vi "main_ctrl.vi"(8 "error in":errorcluster) -> (0 "error out":errorcluster caption="Error")   [LabVIEW 2013]
uses:
  <vilib>/Rock Robotics/WPI/DriverStation/WPI_DriverStationRobotMode2.ctl
  typedefs/fg_typedef.ctl
  typedefs/vision enable.ctl
  typedefs/vision data.ctl
  typedefs/subStates.ctl
  typedefs/singleUseSubstate.ctl
  <vilib>/Rock Robotics/WPI/Solenoid/WPI_SolenoidValue.ctl
  <vilib>/Rock Robotics/WPI/Compressor/WPI_CompressorGetSetRefNum.vi
  <vilib>/Rock Robotics/WPI/RobotDrive/WPI_RobotDriveGetSetRefNum.vi
  <vilib>/Rock Robotics/WPI/Solenoid/WPI_SolenoidSetEnum.vi
  <vilib>/Rock Robotics/WPI/RobotDrive/WPI_RobotDriveArcadeDrive_Standard(NoSaturation).vi
panel:
  out "Robot Mode":T1
  out "Vision SPI":u32
  out "Vision IPS":dbl
  out "Main IPS":dbl
  out "Main SPI":u32
  # "MAIN CONTROL"
  # "holds robot control code - dual parallel state machine"
  # "SPI: milliseconds per iteration\nIPS: iterations per second"
  # "need to incorporate cancel commands"
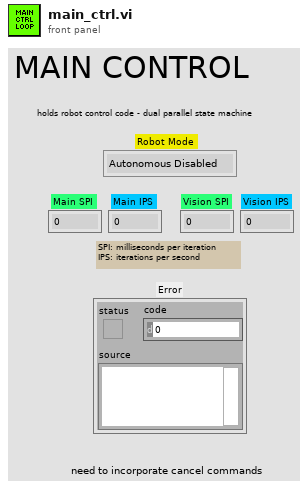
[diagram p1: front panel]
types:
  T1 = typedef "WPI_DriverStationRobotMode2.ctl" = enum16{"Autonomous Disabled", "Autonomous Enabled", "Teleop Disabled", "Teleop Enabled", "Timeout", "Finish", "Test Disabled", "Test Enabled"}
  T2 = typedef "vision data.ctl" = cluster{"x":dbl, "y":dbl, "area":dbl, "width":dbl, "height":dbl, "Hot Goal Present?":bool, "distance":dbl}
  T3 = typedef "vision enable.ctl" = enum16{"Enable", "Disable", "Stop"}
  T4 = typedef "fg_typedef.ctl" = enum16{"Get", "Set"}
  T5 = typedef "WPI_RobotDriveDevRef.ctl" = cluster{"DevStatus":errorcluster, "Motors[]":T6[], "Square Inputs":bool, "Max Output":dbl, "Isochronous":bool}
  T6 = typedef "WPI_MotorControlDeviceRef.ctl" = cluster{"DeviceStatus":errorcluster, "Type":enum16{"PWM", "CAN"}, "PWM":cluster{"Digital Module":T7, "PWM Channel":T8, "DeadBand":T9}, "CAN":cluster{"Device Number":u8, "Control Mode":T10, "Semaphore":T11, "Max Vout":dbl}, "Invert":bool, "TransformRef":T12, "InvTransformRef":T12}
  T7 = typedef "FPGA_TypedefDigitalModule.ctl" = enum16{"Digital Module 1", "Digital Module 2"}
  T8 = typedef "FPGA_DIOPWMChannel.ctl" = enum8{"PWM 1", "PWM 2", "PWM 3", "PWM 4", "PWM 5", "PWM 6", "PWM 7", "PWM 8", "PWM 9", "PWM 10", "Invalid"}
  T9 = typedef "WPI_PWMDeadband.ctl" = cluster{"Name":string, "maxPositivePwm":i32, "minPositivePwm":i32, "centerPwm":i32, "maxNegativePwm":i32, "minNegativePwm":i32, "angularRange":u16}
  T10 = typedef "WPI_CANJaguar_ControlMode.ctl" = enum8{"Percent VBus", "Current", "Speed", "Position", "Voltage"}
  T11 = typedef "Semaphore RefNum" = refnum<k1>
  T12 = typedef "WPI_PWMTransform_ConPane.ctl" = refnum<vi>
  T13 = typedef "WPI_SolenoidDevRef.ctl" = cluster{"DevStatus":errorcluster, "Solenoid Module":T14, "Forward Solenoid Channel":T15, "Reverse Solenoid Channel":T15}
  T14 = typedef "FPGA_TypedefSolenoidModule.ctl" = enum16{"Solenoid Module 1", "Solenoid Module 2"}
  T15 = typedef "WPI_SolenoidChannel.ctl" = enum8{"Solenoid 1", "Solenoid 2", "Solenoid 3", "Solenoid 4", "Solenoid 5", "Solenoid 6", "Solenoid 7", "Solenoid 8", "Invalid"}
  T16 = typedef "WPI_CompressorDevRef.ctl" = cluster{"DevStatus":errorcluster, "DigitalInputDevRef":T17, "RelayDevRef":T19}
  T17 = typedef "WPI_DigitalInputDevRef.ctl" = cluster{"DevStatus":errorcluster, "DIO Channel":T18, "Digital Module":T7}
  T18 = typedef "FPGA_DIOChannel.ctl" = enum8{"DIO 1", "DIO 2", "DIO 3", "DIO 4", "DIO 5", "DIO 6", "DIO 7", "DIO 8", "DIO 9", "DIO 10", "DIO 11", "DIO 12", "DIO 13", "DIO 14", "Invalid"}
  T19 = typedef "WPI_RelayDevRef.ctl" = cluster{"DevStatus":errorcluster, "Relay Channel":T20, "Digital Module":T7, "Relay Direction":T21}
  T20 = typedef "FPGA_DIORelayChannel.ctl" = enum8{"Relay 1", "Relay 2", "Relay 3", "Relay 4", "Relay 5", "Relay 6", "Relay 7", "Relay 8", "Invalid"}
  T21 = typedef "WPI_RelayDirection.ctl" = enum16{"Both directions", "Forward only", "Reverse only"}
  T22 = typedef "WPI_CameraDevRef.ctl" = cluster{"Camera Address":string, "CameraStatus":errorcluster, "Acquire Image Notifier":refnum<notifier>}
  T23 = typedef "IMAQ Image.ctl" = refnum<image>
  T24 = typedef "WPI_SolenoidValue.ctl" = enum16{"Off", "On", "Forward", "Reverse"}
  T25 = typedef "singleUseSubstate.ctl" = enum16{"null", "wait", "shift high", "shift low"}
  T26 = typedef "WPI_DriverStationDerivedRobotMode.ctl" = enum16{"Init", "Execute", "Stop"}
  T27 = typedef "subStates.ctl" = enum16{"null", "wait", "driver control", "auto", "manual override", "hold position", "rotate", "pickup", "pass", "load", "goto shoot", "shoot", "cancel", "end"}
  T28 = typedef "Loop 2 Datatype.ctl" = cluster{"State":T27, "Waiting Loop":i32, "State to Wait For":i32, "Loop ID":i32, "Exit Value":i32, "Joystick Y":dbl, "Tune Speed":dbl}
  T29 = typedef "Loop 1 Datatype.ctl" = cluster{"State":T27, "Waiting Loop":i32, "State to Wait For":i32, "Loop ID":i32, "Exit Value":i32}
  T30 = typedef "Loop 3 Datatype.ctl" = cluster{"State":T27, "Waiting Loop":i32, "State to Wait For":i32, "Loop ID":i32, "Exit Value":i32, "Joystick Y":dbl, "Joystick Z":dbl}
  T31 = typedef "Loop 0 Datatype.ctl" = cluster{"State":T27, "Waiting Loop":i32, "State to Wait For":i32, "Loop ID":i32, "Exit Value":i32, "X Axis":dbl, "Y Axis":dbl, "Z Axis":dbl}
  T32 = typedef "Loop 4 Datatype.ctl" = cluster{"State":T27, "Waiting Loop":i32, "State to Wait For":i32, "Loop ID":i32, "Exit Value":i32}
  T33 = cluster{"Vision mSPI":u32, "Main mSPI":u32, "Dash mSPI":u32}
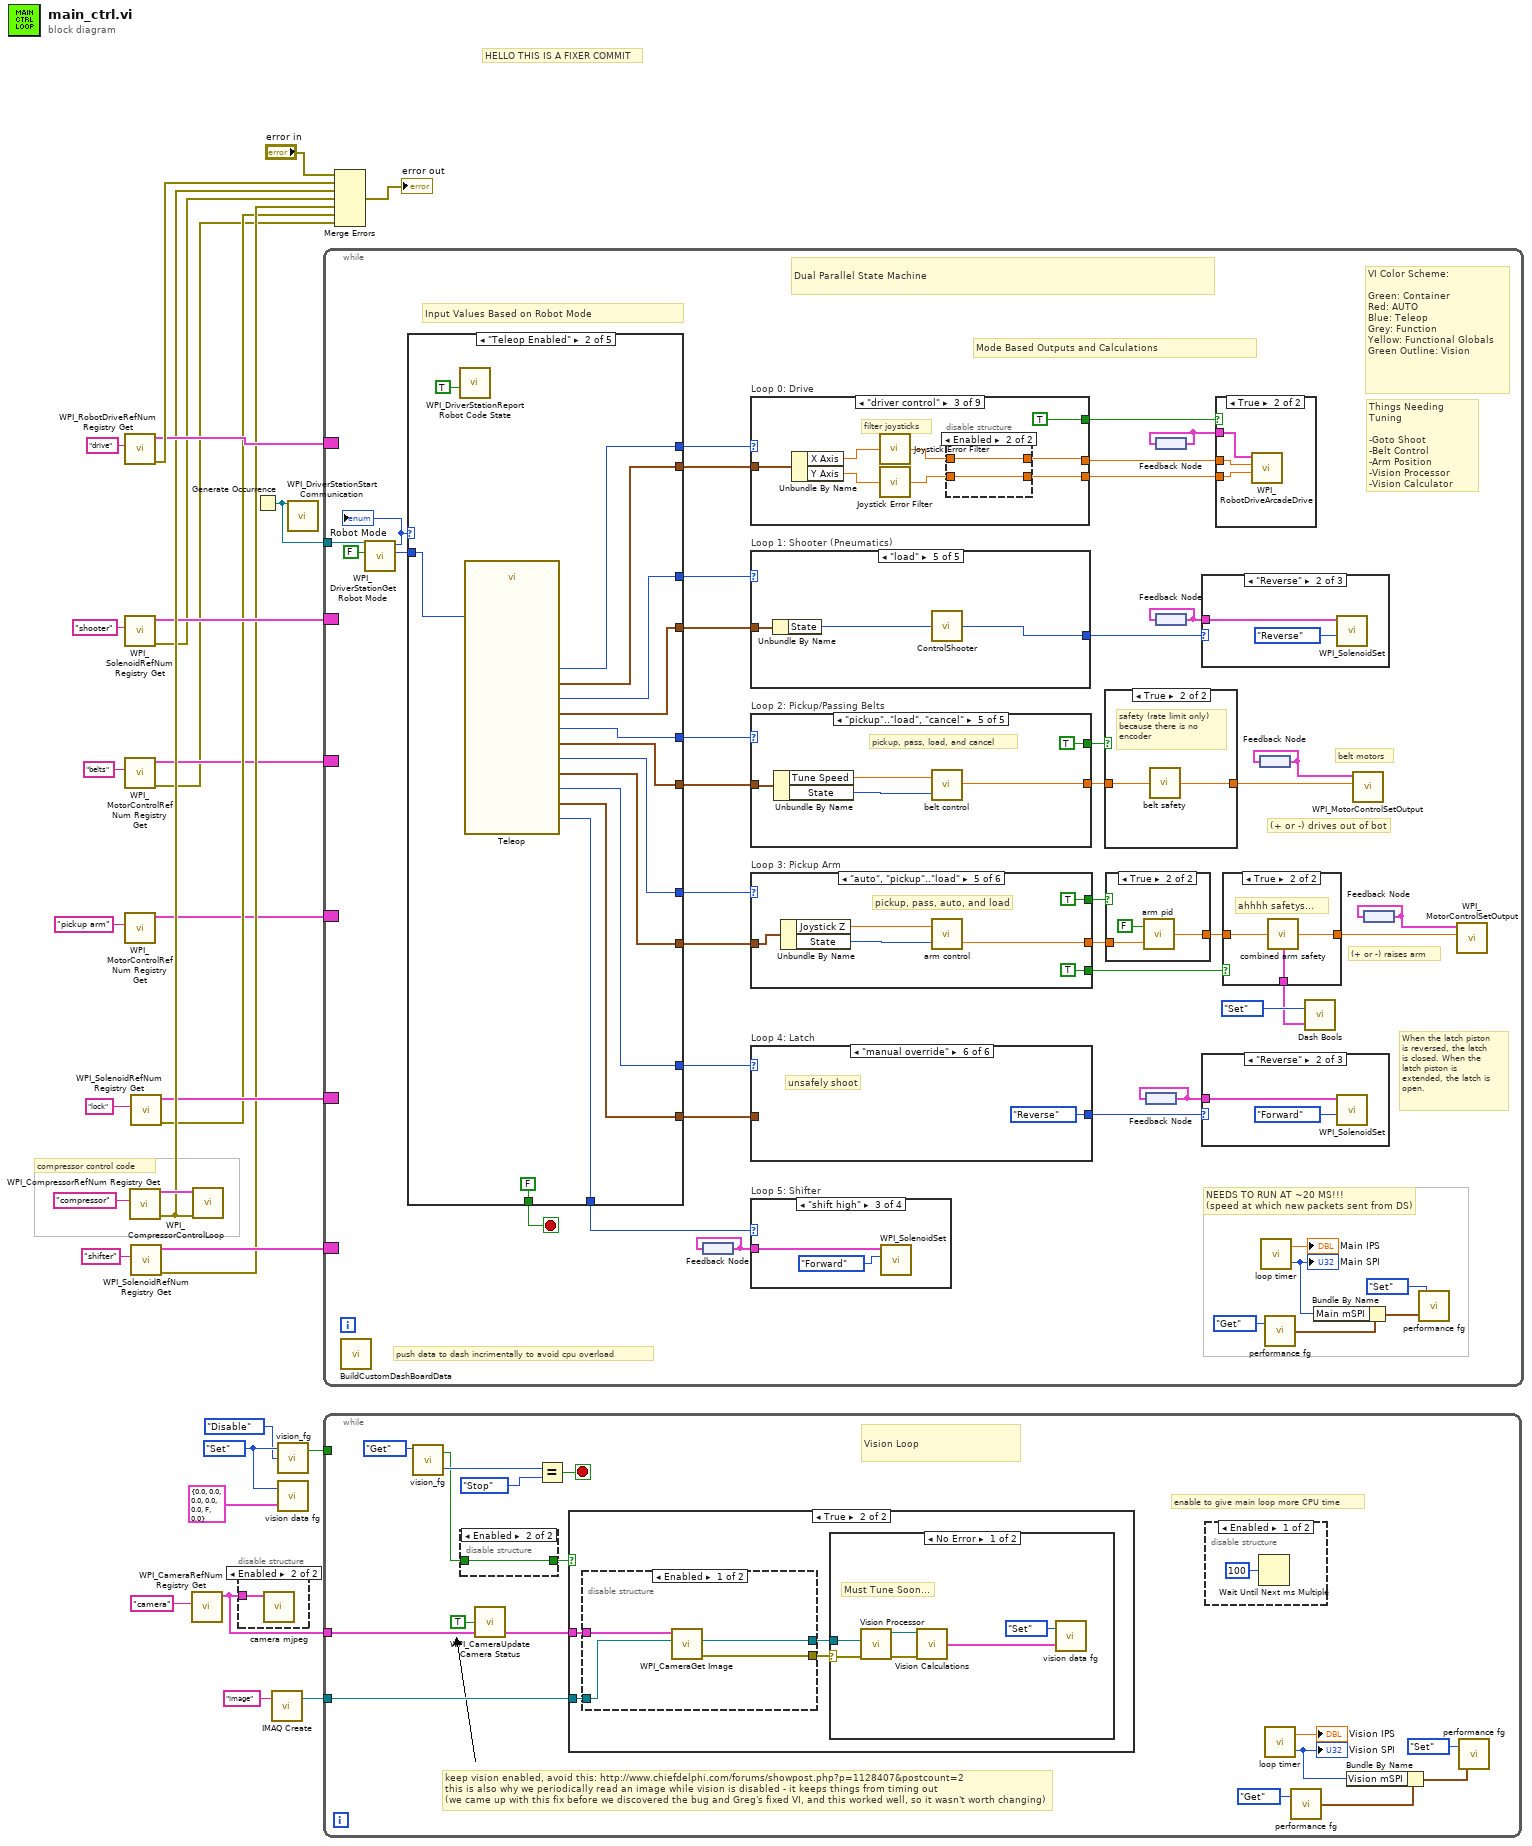
[diagram p0: block diagram]
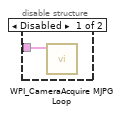
[diagram p2: hidden frame]
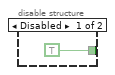
[diagram p3: hidden frame]
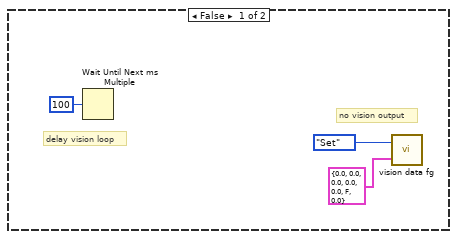
[diagram p5: hidden frame]
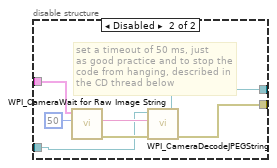
[diagram p7: hidden frame]
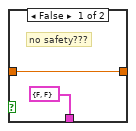
[diagram p9: hidden frame]
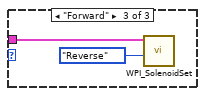
[diagram p12: hidden frame]
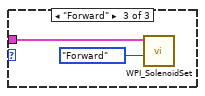
[diagram p14: hidden frame]
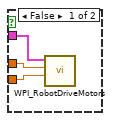
[diagram p15: hidden frame]
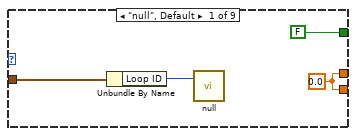
[diagram p16: hidden frame]
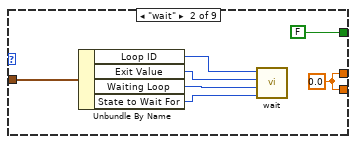
[diagram p17: hidden frame]
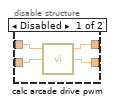
[diagram p18: hidden frame]
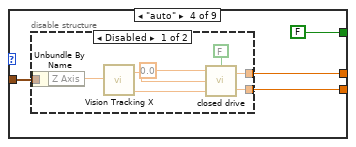
[diagram p19: hidden frame]
diagram:
  w19 = fg_typedef."Set" ("Enum")
  # "compressor control code"
  # "HELLO THIS IS A FIXER COMMIT"
  n1 = call <vilib>:"WPI_RobotDriveRefNum Registry Get.vi"("refnum name"="drive") -> ("error out"=w28:errorcluster, "RobotDriveDevRef"=w26:T5)  [unwired: 9 in]
  n2 = call <vilib>:"WPI_SolenoidRefNum Registry Get.vi"("refnum name"="shooter") -> ("error out"=w7:errorcluster, "SolenoidDevRef"=w11:T13)  [unwired: 9 in]
  n3 = call <vilib>:"WPI_MotorControlRefNum Registry Get.vi"("refnum name"="belts") -> ("error out"=w3:errorcluster, "MotorControlDevRef"=w5:T6)  [unwired: 9 in]
  n4 = call <vilib>:"WPI_MotorControlRefNum Registry Get.vi"("refnum name"="pickup arm") -> ("MotorControlDevRef"=w1:T6)  [unwired: 9 in, 1 out]
  n5 = call <vilib>:"WPI_CompressorRefNum Registry Get.vi"("refnum name"="compressor") -> ("error out"=w22:errorcluster, "CompressorDevRef"=w25:T16)  [unwired: 9 in]
  n6 = call <vilib>:"WPI_SolenoidRefNum Registry Get.vi"("refnum name"="lock") -> ("error out"=w6:errorcluster, "SolenoidDevRef"=w9:T13)  [unwired: 9 in]
  n7 = call <vilib>:"WPI_SolenoidRefNum Registry Get.vi"("refnum name"="shifter") -> ("error out"=w8:errorcluster, "SolenoidDevRef"=w24:T13)  [unwired: 9 in]
  n8 = call <vilib>:"WPI_CameraRefNum Registry Get.vi"("refnum name"="camera") -> ("CameraDevRef"=w16:T22)  [unwired: 9 in, 1 out]
  n9 = call <vilib>:"WPI_CompressorControlLoop.vi"("error in (no error)"=w22, "CompressorDevRef"=w25) -> ()  [unwired: 10 in]
  n10 = disable-structure shown="Enabled" {
    disable-tunnel: w16 -> [w32 w33]
    frame Disabled {
      n11 = call <vilib>:"WPI_CameraAcquire MJPG Loop.vi"("CameraDevRef"=w32) -> ()  [unwired: 11 in]
    }
    frame Enabled {
      n12 = call "camera mjpeg.vi"("CameraDevRef"=w33) -> ()  [unwired: 11 in]
    }
  }
  n13 = Generate Occurrence() -> (w14:refnum<k4>)
  n14 = call "IMAQ Create"("Image Name"="image") -> ("New Image"=w21:T23)  [unwired: 4 in, 1 out]
  n15 = call "vision_fg.vi"("Action"=vision_enable."Disable", "Menu"=w19) -> ("Enabled?"=w20:bool)  [unwired: 1 in, 1 out]
  n16 = call "vision data fg.vi"("Input"=T2 {"x"=0.0, "y"=0.0, "area"=0.0, "width"=0.0, "height"=0.0, "Hot Goal Present?"=FALSE, "distance"=0.0} ("Cluster"), "Menu"=w19) -> ()  [unwired: 1 out]
  n17 = call <vilib>:"WPI_DriverStationStart Communication.vi"("occurrence"=w14) -> ()  [unwired: 11 in]
  n18 = while {
    tunnel: w14 -> [w52]
    border: w26 -> [_]
    border: w24 -> [_]
    border: w11 -> [_]
    border: w9 -> [_]
    border: w5 -> [_]
    border: w1 -> [_]
    stop <- w73 stop-if-true
    # "When the latch piston\nis reversed, the latch\nis closed. When the\nlatch piston is\nextended, the latch is\nopen."
    # "push data to dash incrimentally to avoid cpu overload"
    # "Things Needing Tuning\n\n-Goto Shoot\n-Belt Control\n-Arm Position\n-Vision Processor\n-Vision Calculator"
    # "(+ or -) raises arm"
    # "(+ or -) drives out of bot"
    # "belt motors"
    # "VI Color Scheme:\n\nGreen: Container\nRed: AUTO\nBlue: Teleop\nGrey: Function\nYellow: Functional Globals\nGreen Outline: Vision"
    # "Input Values Based on Robot Mode"
    # "Mode Based Outputs and Calculations"
    # "NEEDS TO RUN AT ~20 MS!!!\n(speed at which new packets sent from DS)"
    # "Dual Parallel State Machine"
    n19 = call "BuildCustomDashBoardData.vi"() -> ()  [unwired: 12 in]
    n20 = call <vilib>:"WPI_DriverStationGet Robot Mode.vi"("Finish"=FALSE, "DS Occurrence"=w52) -> ("Call Context"=w51:T26, "Robot Mode"=w50:T1)  [unwired: 8 out]
    "Robot Mode" <- w50
    n21 = case shown="\"Teleop Enabled\"" w50 {
      tunnel: [w267 w284 w286 w292 w298] -> w54
      tunnel: w51 -> [w258 w280 _ _ _]
      tunnel: [w265 w283 w286 w292 w298] -> w75
      tunnel: [w259 w281 singleUseSubstate."null" ("SubState 5") singleUseSubstate."null" ("SubState 5") singleUseSubstate."null" ("SubState 5")] -> w74
      tunnel: [FALSE FALSE FALSE FALSE TRUE] -> w73
      tunnel: [w269 w279 w286 w292 w298] -> w66
      tunnel: [w268 w278 _ _ _] -> w67
      tunnel: [w266 w277 _ _ _] -> w65
      tunnel: [w264 w276 _ _ _] -> w64
      tunnel: [w262 w275 _ _ _] -> w62
      tunnel: [w260 w274 _ _ _] -> w61
      tunnel: [w261 w273 w286 w292 w298] -> w60
      tunnel: [w263 w272 w286 w292 w298] -> w59
      frame "Autonomous Enabled" {
        n22 = call <vilib>:"WPI_DriverStationReport Robot Code State.vi"("Autonomous"=TRUE) -> ()  [unwired: 10 in, 1 out]
        n23 = call "Autonomous.vi"("Call Context"=w258) -> ("SubState 2"=w265:T27, "Loop 2 Data"=w264:T28, "SubState 1"=w267:T27, "Loop 1 Data"=w266:T29, "Loop 3 Data"=w262:T30, "SubState 0"=w269:T27, "SubState 3"=w263:T27, "Loop 0 Data"=w268:T31, "Loop 4 Data"=w260:T32, "SubState 4"=w261:T27, "SubState 5"=w259:T25)
      }
      frame "Teleop Enabled" {
        n24 = call <vilib>:"WPI_DriverStationReport Robot Code State.vi"("TeleOp"=TRUE) -> ()  [unwired: 10 in, 1 out]
        n25 = call "Teleop.vi"("Call Context"=w280) -> ("SubState 3"=w272:T27, "SubState 4"=w273:T27, "SubState 5"=w281:T25, "Loop 3 Data"=w275:T30, "Loop 4 Data"=w274:T32, "SubState 0"=w279:T27, "Loop 1 Data"=w277:T29, "Loop 0 Data"=w278:T31, "SubState 1"=w284:T27, "Loop 2 Data"=w276:T28, "SubState 2"=w283:T27)  [unwired: 8 in]
      }
      frame "Autonomous Disabled", "Teleop Disabled", "Timeout" {
        w286 = subStates."null" ("SubState 0")
        # "set all loops to null"
        # "make sure to disable vision\nwe don't need it here"
        # "robot disabled, timeout"
        n26 = call <vilib>:"WPI_DriverStationReport Robot Code State.vi"("Disabled"=TRUE) -> ()  [unwired: 10 in, 1 out]
        n27 = call "vision_fg.vi"("Action"=vision_enable."Disable", "Menu"=fg_typedef."Set") -> ()  [unwired: 1 in, 2 out]
      }
      frame "Test Disabled", "Test Enabled" {
        w292 = subStates."null" ("SubState 0")
        # "set all loops to null"
        # "make sure to disable vision\nwe don't need it here"
        # "test, unused"
        n28 = call <vilib>:"WPI_DriverStationReport Robot Code State.vi"("Test"=TRUE) -> ()  [unwired: 10 in, 1 out]
        n29 = call "vision_fg.vi"("Action"=vision_enable."Disable", "Menu"=fg_typedef."Set") -> ()  [unwired: 1 in, 2 out]
      }
      frame "Finish" {
        w298 = subStates."end"  # Stop All Loops
        # "stop the while loop"
        # "stop DS comms"
        # "stop vision loop"
        n30 = call <vilib>:"WPI_DriverStationStop Communication.vi"("StopCommunication"=TRUE) -> ()  [unwired: 10 in, 1 out]
        n31 = call "vision_fg.vi"("Action"=vision_enable."Stop", "Menu"=fg_typedef."Set") -> ()  [unwired: 1 in, 2 out]
      }
    }
    n32 = feedback #1() -> (w63:T13)
    n33 = feedback-in #1(w63) -> ()
    n34 = case "Loop 0: Drive" shown="\"driver control\"" w66 {
      tunnel: w67 -> [w105 w109 w121 w128 w145 w152 _ _ w168]
      tunnel: [w103 w107 w119 w130 w142 w154 w157 w162 w164] -> w57
      tunnel: [w103 w107 w118 w129 w141 w153 w156 w162 w163] -> w56
      tunnel: [FALSE FALSE TRUE FALSE FALSE FALSE FALSE FALSE FALSE] -> w58
      frame "null", Default {
        w103 = 0.0 ("X Axis")
        n35 = Unbundle By Name(w105) -> ("Loop ID"=w106:i32)
        n36 = call "null.vi"("This Loop ID"=w106) -> ()  [unwired: 2 in]
      }
      frame "wait" {
        w107 = 0.0 ("X Axis")
        n37 = Unbundle By Name(w109) -> ("Loop ID"=w113:i32, "Exit Value"=w112:i32, "Waiting Loop"=w111:i32, "State to Wait For"=w110:i32)
        n38 = call "wait.vi"("State to wait for"=w110, "Waiting Loop ID"=w111, "time (ms)"=w112, "Current Loop ID"=w113) -> ()  [unwired: 1 out]
      }
      frame "driver control" {
        # "filter joysticks"
        n39 = Unbundle By Name(w121) -> ("X Axis"=w114:dbl, "Y Axis"=w117:dbl)
        n40 = call "Joystick Error Filter.vi"("Axis"=w114) -> ("Filtered Axis"=w115:dbl)
        n41 = call "Joystick Error Filter.vi"("Axis"=w117) -> ("Filtered Axis"=w116:dbl)
        n42 = disable-structure shown="Enabled" {
          disable-tunnel: w115 -> [w125 w127]
          disable-tunnel: w116 -> [w124 w126]
          disable-tunnel: [w123 w127] -> w119
          disable-tunnel: [w122 w126] -> w118
          frame Disabled {
            n43 = call "calc arcade drive pwm.vi"("Y axis value"=w124, "X axis value"=w125) -> ("Right Speed"=w122:dbl, "Left Speed"=w123:dbl)  [unwired: 1 in, 1 out]
          }
          frame Enabled {
          }
        }
      }
      frame "auto" {
        n44 = disable-structure shown="Disabled" {
          disable-tunnel: [w139 _] -> w130
          disable-tunnel: [w138 _] -> w129
          disable-tunnel: w128 -> [w134 _]
          frame Disabled {
            n45 = Unbundle By Name(w134) -> ("Z Axis"=w132:dbl)
            n46 = call "Vision Tracking X.vi"("Tweak"=w132) -> ("right speed"=w133:dbl, "left speed"=w136:dbl)
            n47 = call "closed drive.vi"("Acrade Drive?"=FALSE, "Y axis value (Left)"=w136, "X axis value (Right)"=w133, "Threshold (.4)"=0.0 ("Threshold")) -> ("right"=w138:dbl, "left"=w139:dbl)
          }
          frame Enabled {
            # "rotates toward target"
            # "not in use this year"
          }
        }
      }
      frame "hold position" {
        n48 = Unbundle By Name(w145) -> ("X Axis"=w144:dbl, "Y Axis"=w143:dbl)
        n49 = call "closed drive.vi"("Acrade Drive?"=TRUE, "Y axis value (Left)"=w143, "X axis value (Right)"=w144) -> ("right"=w141:dbl, "left"=w142:dbl)  [unwired: 1 in]
      }
      frame "rotate" {
        # "use these to carry actual information because this is\nfor autonomous only so there will not be joystick input"
        n50 = Unbundle By Name(w152) -> ("X Axis"=w151:dbl, "Y Axis"=w150:dbl)
        n51 = call "rotate.vi"("Angle"=w151, "Rate"=w150) -> ("finished?"=w147:bool, "left speed"=w154:dbl, "right speed"=w153:dbl)
        n52 = call "states FG.vi"("exit in"=w147, "menu (get)"=enum16{"set", "get"}."set", "Loop ID"=0) -> ()  [unwired: 5 in, 4 out]
      }
      frame "goto shoot" {
        # "consider implimenting closed hold with drive"
        n53 = call "vision data fg.vi"("Menu"=fg_typedef."Get") -> ("Output"=w158:T2)  [unwired: 1 in]
        n54 = call "goto location.vi"("Image Data"=w158) -> ("left speed"=w157:dbl, "right speed"=w156:dbl)
      }
      frame "end" {
        w162 = 0.0 ("X Axis")
      }
      frame "manual override" {
        n55 = Unbundle By Name(w168) -> ("X Axis"=w167:dbl, "Y Axis"=w166:dbl)
        n56 = expression code="x/2"(w167) -> (w164:dbl)
        n57 = expression code="x/2"(w166) -> (w163:dbl)
      }
    }
    n58 = case "Loop 1: Shooter (Pneumatics)" shown="\"load\"" w54 {
      tunnel: w65 -> [w244 w247 _ _ w256]
      tunnel: [WPI_SolenoidValue."Off" ("Value") WPI_SolenoidValue."Off" ("Value") WPI_SolenoidValue."Off" ("Value") WPI_SolenoidValue."Off" ("Value") w254] -> w49
      frame "null", Default {
        n59 = Unbundle By Name(w244) -> ("Loop ID"=w245:i32)
        n60 = call "null.vi"("This Loop ID"=w245) -> ()  [unwired: 2 in]
      }
      frame "wait" {
        n61 = Unbundle By Name(w247) -> ("Loop ID"=w251:i32, "Exit Value"=w250:i32, "Waiting Loop"=w249:i32, "State to Wait For"=w248:i32)
        n62 = call "wait.vi"("State to wait for"=w248, "Waiting Loop ID"=w249, "time (ms)"=w250, "Current Loop ID"=w251) -> ()  [unwired: 1 out]
      }
      frame "driver control" {
      }
      frame "manual override" {
      }
      frame "load" {
        n63 = Unbundle By Name(w256) -> ("State"=w255:T27)
        n64 = call "ControlShooter.vi"("State"=w255) -> ("To Shooter\nSolenoid Loop"=w254:T24)
      }
    }
    n65 = case "Loop 2: Pickup/Passing Belts" shown="\"pickup\"..\"load\", \"cancel\"" w75 {
      tunnel: w64 -> [w222 w225 w233 w237 w242]
      tunnel: [0.0 ("output") 0.0 ("output") w231 w235 w239] -> w37
      tunnel: [FALSE FALSE TRUE FALSE TRUE] -> w38
      frame "null", Default {
        n66 = Unbundle By Name(w222) -> ("Loop ID"=w221:i32)
        n67 = call "null.vi"("This Loop ID"=w221) -> ()  [unwired: 2 in]
      }
      frame "wait" {
        n68 = Unbundle By Name(w225) -> ("Loop ID"=w229:i32, "Exit Value"=w228:i32, "Waiting Loop"=w227:i32, "State to Wait For"=w226:i32)
        n69 = call "wait.vi"("State to wait for"=w226, "Waiting Loop ID"=w227, "time (ms)"=w228, "Current Loop ID"=w229) -> ()  [unwired: 1 out]
      }
      frame "driver control" {
        n70 = Unbundle By Name(w233) -> ("Joystick Y"=w230:dbl)
        n71 = call "Joystick Error Filter.vi"("Axis"=w230) -> ("Filtered Axis"=w231:dbl)
      }
      frame "manual override" {
        n72 = Unbundle By Name(w237) -> ("Joystick Y"=w236:dbl)
        n73 = expression code="x/2"(w236) -> (w235:dbl)
      }
      frame "pickup".."load", "cancel" {
        # "pickup, pass, load, and cancel"
        n74 = Unbundle By Name(w242) -> ("Tune Speed"=w241:dbl, "State"=w240:T27)
        n75 = call "belt control.vi"("State"=w240, "Joystick Z"=w241) -> ("output"=w239:dbl)
      }
    }
    n76 = case "Loop 3: Pickup Arm" shown="\"auto\", \"pickup\"..\"load\"" w59 {
      tunnel: w62 -> [w187 w191 w199 w205 w211 _]
      tunnel: [FALSE FALSE FALSE FALSE TRUE TRUE] -> w43
      tunnel: [0.0 ("output") 0.0 ("output") w196 w203 w207 0.0 ("setpoint")] -> w42
      tunnel: [TRUE TRUE TRUE FALSE TRUE TRUE] -> w41
      frame "null", Default {
        n77 = Unbundle By Name(w187) -> ("Loop ID"=w186:i32)
        n78 = call "null.vi"("This Loop ID"=w186) -> ()  [unwired: 2 in]
      }
      frame "wait" {
        n79 = Unbundle By Name(w191) -> ("Loop ID"=w195:i32, "Exit Value"=w194:i32, "Waiting Loop"=w193:i32, "State to Wait For"=w192:i32)
        n80 = call "wait.vi"("State to wait for"=w192, "Waiting Loop ID"=w193, "time (ms)"=w194, "Current Loop ID"=w195) -> ()  [unwired: 1 out]
      }
      frame "driver control" {
        n81 = Unbundle By Name(w199) -> ("Joystick Y"=w197:dbl)
        n82 = call "Joystick Error Filter.vi"("Axis"=w197) -> ("Filtered Axis"=w196:dbl)
      }
      frame "manual override" {
        n83 = Unbundle By Name(w205) -> ("Joystick Y"=w204:dbl)
        n84 = expression code="x/2"(w204) -> (w203:dbl)
      }
      frame "auto", "pickup".."load" {
        # "pickup, pass, auto, and load"
        n85 = Unbundle By Name(w211) -> ("Joystick Z"=w209:dbl, "State"=w208:T27)
        n86 = call "arm control.vi"("State"=w208, "Z Axis (Tuning)"=w209) -> ("setpoint"=w207:dbl)
      }
      frame "hold position" {
        # "it just re-initalized, so 0 means don't move"
      }
    }
    n87 = case "Loop 4: Latch" shown="\"manual override\"" w60 {
      tunnel: w61 -> [w171 w173 _ _ _ _]
      tunnel: [WPI_SolenoidValue."Off" ("Value") WPI_SolenoidValue."Off" ("Value") WPI_SolenoidValue."Off" ("Value") w180 WPI_SolenoidValue."Forward" ("Value") WPI_SolenoidValue."Reverse" ("Value")] -> w46
      frame "null", Default {
        n88 = Unbundle By Name(w171) -> ("Loop ID"=w170:i32)
        n89 = call "null.vi"("This Loop ID"=w170) -> ()  [unwired: 2 in]
      }
      frame "wait" {
        n90 = Unbundle By Name(w173) -> ("Loop ID"=w177:i32, "Exit Value"=w176:i32, "Waiting Loop"=w175:i32, "State to Wait For"=w174:i32)
        n91 = call "wait.vi"("State to wait for"=w174, "Waiting Loop ID"=w175, "time (ms)"=w176, "Current Loop ID"=w177) -> ()  [unwired: 1 out]
      }
      frame "driver control" {
      }
      frame "shoot" {
        # "aka disengage latch"
        n92 = call "latch shoot.vi"() -> ("Latch"=w179:T24)
        n93 = call "re-init on shoot.vi"("Relay Value"=w179) -> ("Value"=w180:T24)
      }
      frame "auto" {
        # "aka engage"
      }
      frame "manual override" {
        # "unsafely shoot"
      }
    }
    n94 = case "Loop 5: Shifter" shown="\"shift high\"" w74 {
      tunnel: w63 -> [_ _ w216 w217]
      frame "null", Default {
      }
      frame "wait" {
      }
      frame "shift high" {
        n95 = call-poly <vilib>:"WPI_SolenoidSet.vi"("Value"=WPI_SolenoidValue."Forward", "SolenoidDevRef"=w216) -> ()  [unwired: 8 in, 2 out]
      }
      frame "shift low" {
        n96 = call-poly <vilib>:"WPI_SolenoidSet.vi"("Value"=WPI_SolenoidValue."Reverse", "SolenoidDevRef"=w217) -> ()  [unwired: 8 in, 2 out]
      }
    }
    n97 = case shown="True" w38 {
      tunnel: w37 -> [w77 w79]
      tunnel: [w77 w78] -> w36
      frame False {
        # "no safety"
      }
      frame True {
        # "safety (rate limit only)\nbecause there is no \nencoder"
        n98 = call "belt safety.vi"("Input"=w79) -> ("Safe Output"=w78:dbl)
      }
    }
    n99 = case shown="True" w43 {
      tunnel: w42 -> [w85 w88]
      tunnel: [w85 w86] -> w40
      frame False {
        # "open loop"
      }
      frame True {
        n100 = call "arm pid.vi"("Setpoint"=w88, "Autotune?"=FALSE) -> ("Output"=w86:dbl)
      }
    }
    n101 = feedback #2() -> (w47:T13)
    n102 = feedback-in #2(w47) -> ()
    n103 = feedback #3() -> (w55:T5)
    n104 = feedback-in #3(w55) -> ()
    n105 = feedback #4() -> (w48:T13)
    n106 = feedback-in #4(w48) -> ()
    n107 = case shown="\"Reverse\"" w49 {
      tunnel: w48 -> [_ w93 w95]
      frame "Off", Default {
      }
      frame "Reverse" {
        n108 = call-poly <vilib>:"WPI_SolenoidSet.vi"("Value"=WPI_SolenoidValue."Reverse", "SolenoidDevRef"=w93) -> ()  [unwired: 8 in, 2 out]
      }
      frame "Forward" {
        n109 = call-poly <vilib>:"WPI_SolenoidSet.vi"("Value"=WPI_SolenoidValue."Forward", "SolenoidDevRef"=w95) -> ()  [unwired: 8 in, 2 out]
      }
    }
    n110 = case shown="\"Reverse\"" w46 {
      tunnel: w47 -> [_ w89 w91]
      frame "Off", Default {
      }
      frame "Reverse" {
        n111 = call-poly <vilib>:"WPI_SolenoidSet.vi"("Value"=WPI_SolenoidValue."Forward", "SolenoidDevRef"=w89) -> ()  [unwired: 8 in, 2 out]
      }
      frame "Forward" {
        n112 = call-poly <vilib>:"WPI_SolenoidSet.vi"("Value"=WPI_SolenoidValue."Reverse", "SolenoidDevRef"=w91) -> ()  [unwired: 8 in, 2 out]
      }
    }
    n113 = case shown="True" w58 {
      tunnel: w57 -> [w98 w102]
      tunnel: w56 -> [w97 w101]
      tunnel: w55 -> [w99 w100]
      frame False {
        n114 = call <vilib>:"WPI_RobotDriveMotors.vi"("RightSpeed"=w97, "LeftSpeed"=w98, "RobotDriveDevRef"=w99) -> ()  [unwired: 6 in, 3 out]
      }
      frame True {
        n115 = call-poly <vilib>:"WPI_RobotDriveArcadeDrive.vi"("Y axis value"=w101, "X axis value"=w102, "RobotDriveDevRef"=w100) -> ()  [unwired: 6 in, 3 out]
      }
    }
    n116 = case shown="True" w41 {
      tunnel: w40 -> [w81 w84]
      tunnel: [w81 w83] -> w39
      tunnel: [cluster{"Arm Safety":bool, "Arm Limit":bool} {"Arm Safety"=FALSE, "Arm Limit"=FALSE} ("Input") w82] -> w34
      frame False {
        # "no safety???"
      }
      frame True {
        # "ahhhh safetys..."
        n117 = call "combined arm safety.vi"("Input"=w84) -> ("Safe Output"=w83:dbl, "Safety"=w82:cluster{"Arm Safety":bool, "Arm Limit":bool})  [unwired: 13 in]
      }
    }
    n118 = feedback #5() -> (w45:T6)
    n119 = feedback-in #5(w45) -> ()
    n120 = call "loop timer.vi"() -> ("IPS"=→"Main IPS":dbl, "SPI"=w72:u32)  [unwired: 1 in]
    "Main SPI" <- w72
    n121 = call "performance fg.vi"("Menu"=fg_typedef."Get") -> ("Output"=w69:T33)  [unwired: 1 in]
    n122 = call "Dash Bools.vi"("Input"=w34, "Menu"=fg_typedef."Set") -> ()  [unwired: 1 out]
    n123 = Bundle By Name(cluster=w69, "Main mSPI"=w72) -> (w68:T33)
    n124 = call <vilib>:"WPI_MotorControlSetOutput.vi"("Output"=w36, "MotorControlDevRef"=w45) -> ()  [unwired: 7 in, 3 out]
    n125 = feedback #6() -> (w44:T6)
    n126 = feedback-in #6(w44) -> ()
    n127 = call "performance fg.vi"("Input"=w68, "Menu"=fg_typedef."Set") -> ()  [unwired: 1 out]
    n128 = call <vilib>:"WPI_MotorControlSetOutput.vi"("Output"=w39, "MotorControlDevRef"=w44) -> ()  [unwired: 7 in, 3 out]
  }
  n129 = while {
    tunnel: w21 -> [w317]
    tunnel: w16 -> [w316]
    tunnel: w20 -> [_]
    stop <- w318 stop-if-true
    # "keep vision enabled, avoid this: http://www.chiefdelphi.com/forums/showpost.php?p=1128407&postcount=2\nthis is also why we periodically read an image while vision is disabled - it keeps things from timing out\n(we came up with this fix before we discovered the bug and Greg's fixed VI, and this worked well, so it wasn't worth changing)"
    # "enable to give main loop more CPU time"
    # "Vision Loop"
    n130 = call "vision_fg.vi"("Menu"=fg_typedef."Get" ("Enum")) -> ("State Out"=w312:T3, "Enabled?"=w303:bool)  [unwired: 2 in]
    n131 = disable-structure shown="Enabled" {
      disable-tunnel: [TRUE w320] -> w304
      disable-tunnel: w303 -> [_ w320]
      frame Disabled {
      }
      frame Enabled {
      }
    }
    n132 = call <vilib>:"WPI_CameraUpdate Camera Status.vi"("CameraDevRef In"=w316, "Enable Vision"=TRUE) -> ("CameraDevRef Out"=w315:T22)  [unwired: 3 in]
    n133 = Equal?(x=w312, y=vision_enable."Stop") -> (x = y?=w318:bool)
    n134 = case shown="True" w304 {
      tunnel: w317 -> [_ w328]
      tunnel: w315 -> [_ w327]
      frame False {
        # "no vision output"
        # "delay vision loop"
        n135 = Wait Until Next ms Multiple(millisecond multiple=u32 100) -> ()  [unwired: 1 out]
        n136 = call "vision data fg.vi"("Input"=T2 {"x"=0.0, "y"=0.0, "area"=0.0, "width"=0.0, "height"=0.0, "Hot Goal Present?"=FALSE, "distance"=0.0} ("Cluster"), "Menu"=fg_typedef."Set" ("Enum")) -> ()  [unwired: 1 out]
      }
      frame True {
        n137 = disable-structure shown="Enabled" {
          disable-tunnel: w328 -> [w337 w341]
          disable-tunnel: w327 -> [w338 w343]
          disable-tunnel: [w336 w340] -> w326
          disable-tunnel: [w335 w339] -> w325
          frame Enabled {
            n138 = call <vilib>:"WPI_CameraGet Image.vi"("Image"=w337, "CameraDevRef"=w338) -> ("error out"=w335:errorcluster, "Image Out"=w336:T23)  [unwired: 7 in, 1 out]
          }
          frame Disabled {
            # "set a timeout of 50 ms, just\nas good practice and to stop the \ncode from hanging, described in \nthe CD thread below"
            n139 = call <vilib>:"WPI_CameraWait for Raw Image String.vi"("Timeout in ms (-1)"=50, "CameraDevRef"=w343) -> ("error out"=w345:errorcluster, "String"=w344:string)  [unwired: 3 in, 5 out]
            n140 = call <vilib>:"WPI_CameraDecodeJPEGString.vi"("error in"=w345, "Compressed Image"=w344, "Image In"=w341) -> ("error out"=w339:errorcluster, "Image Out"=w340:T23)  [unwired: 3 out]
          }
        }
        n141 = case shown="No Error" w325 {
          selector: w325 -> [w333 _]
          tunnel: w326 -> [w332 _]
          frame No Error {
            # "Must Tune Soon..."
            n142 = call "Vision Processor.vi"("error in"=w333, "Image In"=w332) -> ("error out"=w330:errorcluster, "Image Out"=w331:T23)  [unwired: 5 in]
            n143 = call "Vision Calculations.vi"("Image In"=w331, "error in"=w330) -> ("Vision Data"=w329:T2)  [unwired: 3 in]
            n144 = call "vision data fg.vi"("Input"=w329, "Menu"=fg_typedef."Set" ("Enum")) -> ()  [unwired: 1 out]
          }
          frame Error {
          }
        }
      }
    }
    n145 = disable-structure shown="Enabled" {
      frame Enabled {
        n146 = Wait Until Next ms Multiple(millisecond multiple=u32 100) -> ()  [unwired: 1 out]
      }
      frame Disabled {
      }
    }
    n147 = call "loop timer.vi"() -> ("IPS"=→"Vision IPS":dbl, "SPI"=w310:u32)  [unwired: 1 in]
    "Vision SPI" <- w310
    n148 = call "performance fg.vi"("Menu"=fg_typedef."Get") -> ("Output"=w308:T33)  [unwired: 1 in]
    n149 = Bundle By Name(cluster=w308, "Vision mSPI"=w310) -> (w307:T33)
    n150 = call "performance fg.vi"("Input"=w307, "Menu"=fg_typedef."Set") -> ()  [unwired: 1 out]
  }
  n151 = Merge Errors("error in", w28, w22, w7, w8, w6, w3) -> (→"error out":errorcluster)
